vi "Robot Global Data.vi"() -> ()   [LabVIEW 2015]
doc: "This global VI can contain as many global variables as you need. Place a control on the panel, give it a good name. To read or write to it from a VI, drag the icon to the diagram of that VI. You can also drag from the project. Click on the node to change which global you access. You shouldn't have multiple locations writing to a global or it will cause a race-condition."
uses:
  <vilib>/Rock Robotics/WPI/Camera/WPI_CameraImageSize.ctl
  <vilib>/Rock Robotics/WPI/DriverStation/WPI_DriverStationRobotMode2.ctl
panel:
  out "Put Arm Bottom":bool
  out "Turn off wheels":bool
  out "Joysticks In Range":bool
  out "ARM GOOD":bool
  out "WHEELS GOOD":bool
  out "Ball Holder Override":bool
  in  "Scaled Vision X":dbl
  in  "Wheel Speed":dbl
  out "FIRE":bool
  out "Shooter Data":T1
  out "Vision In Range":bool
  out "Arm Down":bool
  out "Arm Up":bool
  in  "Shooter Actual Speed (RPM)":dbl
  in  "Shooter Setpoint Speed (RPM)":dbl
  out "Target Detected":bool
  in  "Arm Setpoint":dbl
  out "Vision Tracking Enabled":bool
  in  "Vision Turning Value":dbl
  in  "Pot Value":dbl
  in  "Vision  Y":dbl
  in  "Vision X":dbl
  out "ms to process":u32
  out "Detected Totes":T2(array[cluster]) {"Normalized Rect"."Numeric 5" format="%#_2g"; "Normalized Rect"."Numeric 3" format="%#_2g"; "Normalized Rect"."Numeric 2" format="%#_2g"; "Normalized Rect"."Numeric" format="%#_2g"}
  in  "Starting Arm Value":dbl
  in  "Robot Mode":T3
  in  "image size":T4=enum."320x240"
  in  "Enable Vision":bool
  # "Shooter Arm"
  # "Vision"
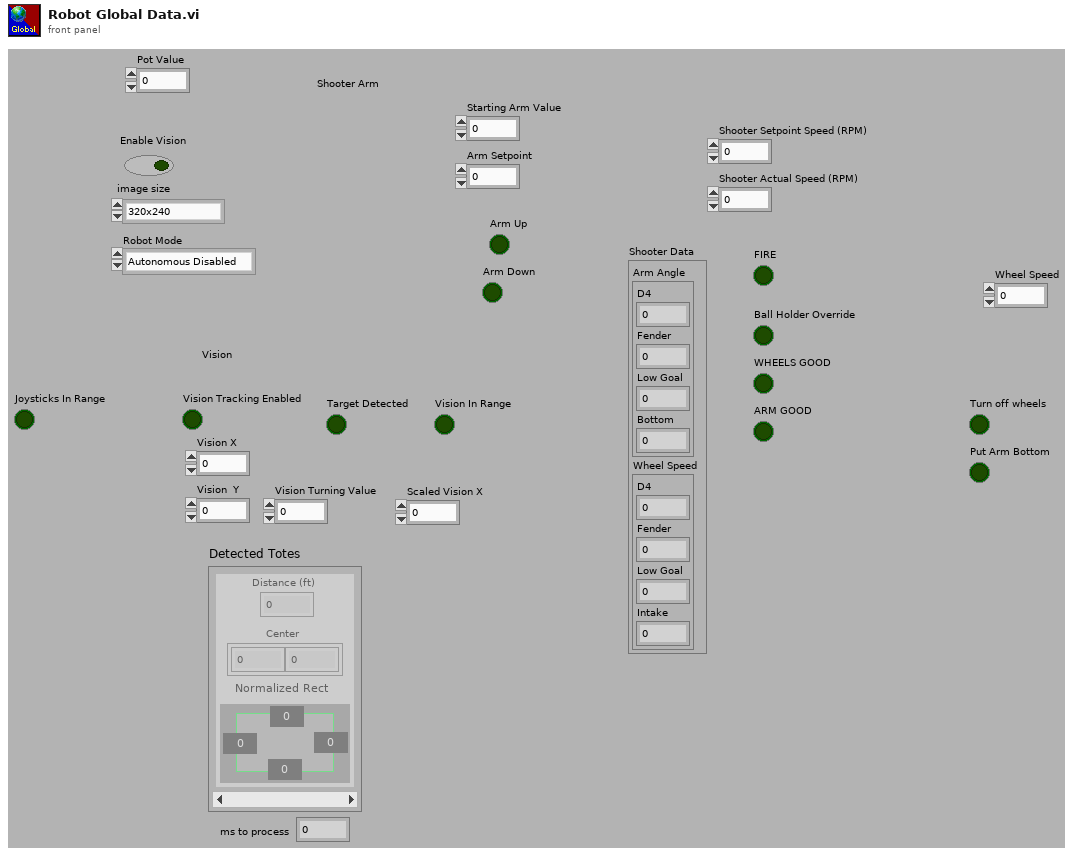
[diagram p1: front panel]
types:
  T1 = cluster{"Arm Angle":cluster{"D4":dbl, "Fender":dbl, "Low Goal":dbl, "Bottom":dbl}, "Wheel Speed":cluster{"D4":dbl, "Fender":dbl, "Low Goal":dbl, "Intake":dbl}}
  T2 = cluster{"Distance (ft)":dbl, "Center":cluster{dbl, dbl}, "Normalized Rect":cluster{"Numeric":dbl, "Numeric 2":dbl, "Numeric 3":dbl, "Numeric 5":dbl}}[]
  T3 = typedef "WPI_DriverStationRobotMode2.ctl" = enum16{"Autonomous Disabled", "Autonomous Enabled", "Teleop Disabled", "Teleop Enabled", "Disconnected", "Finish", "Test Disabled", "Test Enabled", "Emergency Stopped"}
  T4 = typedef "WPI_CameraImageSize.ctl" = enum16{"640x480", "320x240", "160x120", "Custom"}
diagram:
